vi "bartenderprint.vi"(8 "错误输入":errorcluster, 10 "Bartender File Path":string, 11 "PrintString":string) -> (0 "错误输出":errorcluster)   [LabVIEW 2011]
uses:
  Data/Interop.BarTender.dll
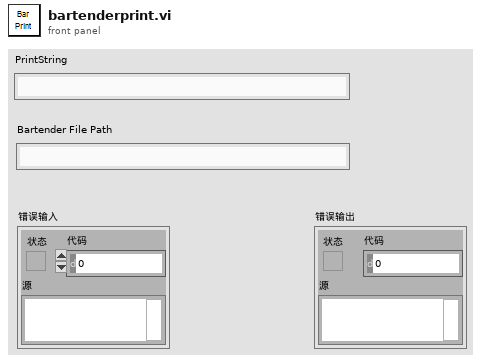
[diagram p1: front panel]
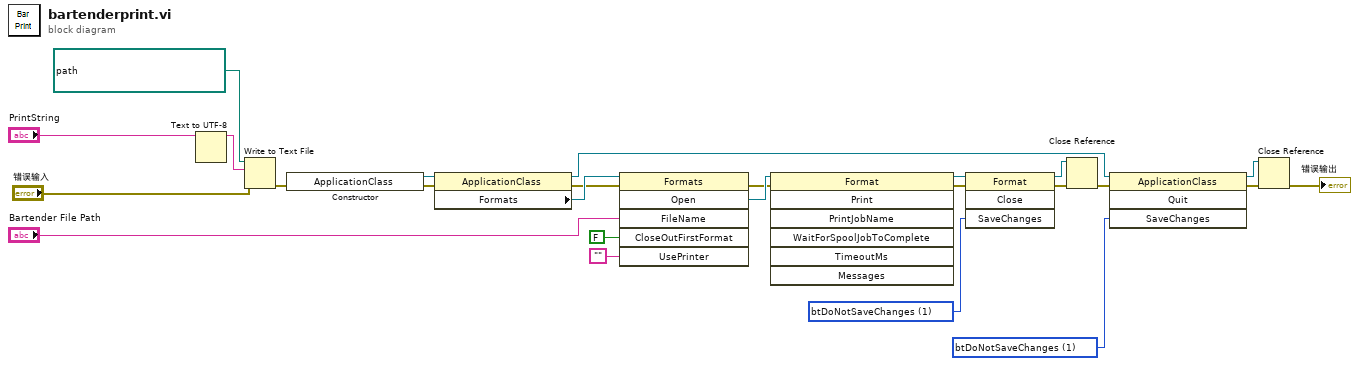
[diagram p0: block diagram]
diagram:
  w9 = 1 items=["btPromptSave", "btDoNotSaveChanges", "btSaveChanges"] ("SaveChanges")
  w11 = 1 items=["btPromptSave", "btDoNotSaveChanges", "btSaveChanges"] ("SaveChanges")
  n1 = Text to UTF-8(11:"PrintString") -> (3:w24:string)  [unwired: 1 in, 1 out]
  n2 = Write to Text File(file (use dialog)=path "C:/Program Files/默认公司名称/Bartender.txt" ("文件（使用对话框）"), text=w24, error in="错误输入") -> (error out=w2:errorcluster)  [unwired: 1 in, 2 out]
  n3 = constructor class="ApplicationClass"(error in=w2) -> (reference out=w22:refnum<k24>, error out=w19:errorcluster)  [unwired: 2 in, 1 out]
  n4 = property class="ApplicationClass"(reference=w22, error in=w19) -> (reference out=w10:refnum<k24>, error out=w18:errorcluster, "Formats"=w21:refnum<k24>)
  n5 = invoke class="Formats" method="Open"(reference=w21, error in=w18, "FileName"="Bartender File Path", "CloseOutFirstFormat"=FALSE, "UsePrinter"="") -> (error out=w17:errorcluster, "Open"=w20:refnum<k24>)  [unwired: 1 in, 4 out]
  n6 = invoke class="Format" method="Print"(reference=w20, error in=w17) -> (reference out=w12:refnum<k24>, error out=w13:errorcluster)  [unwired: 5 in, 5 out]
  n7 = invoke class="Format" method="Close"(reference=w12, error in=w13, "SaveChanges"=w11) -> (reference out=w7:refnum<k24>, error out=w8:errorcluster)  [unwired: 1 in, 2 out]
  n8 = Close Reference(reference=w7, error in (no error)=w8) -> (error out=w6:errorcluster)
  n9 = invoke class="ApplicationClass" method="Quit"(reference=w10, error in=w6, "SaveChanges"=w9) -> (reference out=w4:refnum<k24>, error out=w5:errorcluster)  [unwired: 1 in, 2 out]
  n10 = Close Reference(reference=w4, error in (no error)=w5) -> (error out=→"错误输出":errorcluster)
